vi "Update Waveform Array.vi"(8 "error in (no error)":errorcluster caption="错误输入（无错误）", 10 "new waveform array":waveform(dbl)[](array[waveform]) caption="新波形数组", 11 "original waveform array":waveform(dbl)[](array[waveform]) caption="原波形数组") -> (0 "error out":errorcluster caption="错误输出", 2 "min duration":dbl caption="最小时长", 3 "updated wavefrom array":waveform(dbl)[](array[waveform]) caption="更新后波形数组")   [LabVIEW 2015]
uses:
  <vilib>/Waveform/WDTOps.llb/WDT Index Channel DBL.vi
  <vilib>/Waveform/WDTOps.llb/WDT Append Waveforms DBL.vi
  <vilib>/Waveform/WDTOps.llb/WDT Waveform Duration DBL.vi
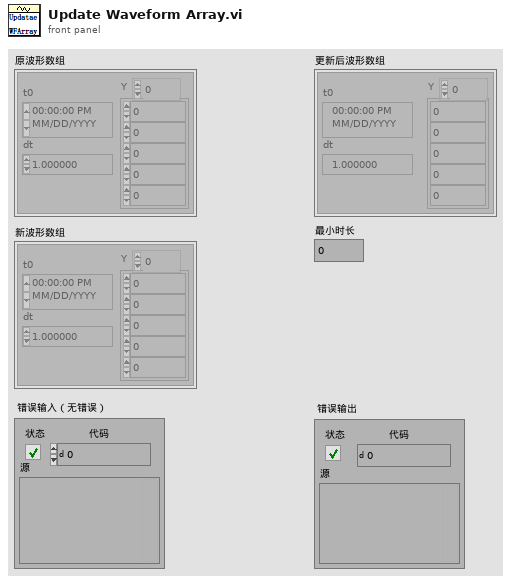
[diagram p1: front panel]
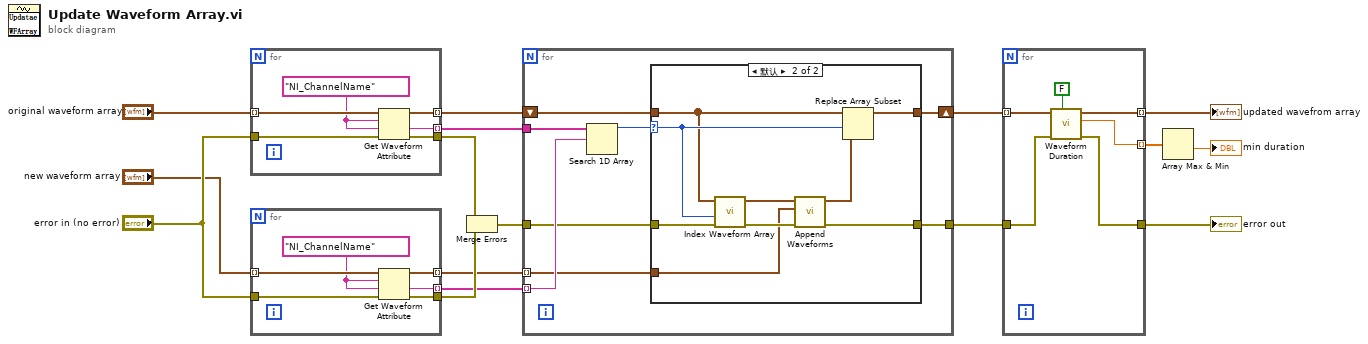
[diagram p0: block diagram]
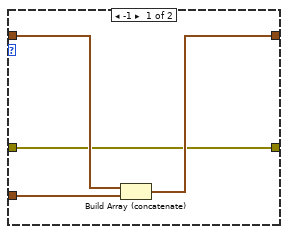
[diagram p2: hidden frame]
diagram:
  n1 = for {
    tunnel: "original waveform array" -> [w22] mode=indexing
    tunnel: "error in (no error)" -> [w21]
    tunnel: [w19] -> w14 mode=indexing
    tunnel: [w18] -> w13 mode=indexing
    tunnel: [w17] -> w11
    w20 = "NI_ChannelName" ("名称")
    n2 = Get Waveform Attribute(4:w21, 5:w20, 6:w20, 7:w22) -> (0:w17:errorcluster, 1:w19:string, 3:w18:waveform(dbl))  [unwired: 1 out]
  }
  n3 = for {
    tunnel: "new waveform array" -> [w28] mode=indexing
    tunnel: "error in (no error)" -> [w27]
    tunnel: [w25] -> w10 mode=indexing
    tunnel: [w24] -> w9 mode=indexing
    tunnel: [w23] -> w12
    w26 = "NI_ChannelName" ("名称")
    n4 = Get Waveform Attribute(4:w27, 5:w26, 6:w26, 7:w28) -> (0:w23:errorcluster, 1:w25:string, 3:w24:waveform(dbl))  [unwired: 1 out]
  }
  n5 = Merge Errors(w11, w12) -> (w8:errorcluster)
  n6 = for {
    tunnel: w14 -> [w36]
    tunnel: w10 -> [w35] mode=indexing
    tunnel: w9 -> [w32] mode=indexing
    shift-right: [w30] -> w7
    shift-left: w13 -> [w31]
    tunnel: w8 -> [w33]
    tunnel: [w29] -> w5
    n7 = Search 1D Array(1D array=w36, element=w35) -> (index of element=w34:i32)  [unwired: 1 in]
    n8 = case shown="默认" w34 {
      selector: w34 -> [_ w45]
      tunnel: w31 -> [w40 w41]
      tunnel: w33 -> [w37 w47]
      tunnel: w32 -> [w39 w46]
      tunnel: [w38 w43] -> w30
      tunnel: [w37 w42] -> w29
      frame -1 {
        n9 = Build Array (concatenate)(w40, w39) -> (w38:waveform(dbl)[])
      }
      frame Default {
        n10 = call-poly <vilib>:"Index Waveform Array.vi"("error in (no error)"=w47, "index"=w45, "waveform array"=w41) -> ("error out"=w48:errorcluster, "waveform"=w49:waveform(dbl))  [unwired: 7 in]
        n11 = call-poly <vilib>:"Append Waveforms.vi"("error in (no error)"=w48, "waveform B"=w46, "waveform A"=w49) -> ("error out"=w42:errorcluster, "waveform out"=w44:waveform(dbl))  [unwired: 7 in]
        n12 = Replace Array Subset(array=w41, new element=w44, index=w45) -> (w43:waveform(dbl)[])
      }
    }
  }
  n13 = for {
    tunnel: w7 -> [w55] mode=indexing
    tunnel: [w54] -> w6 mode=indexing
    tunnel: w5 -> [w53]
    tunnel: [w52] -> w4
    tunnel: [w51] -> w2 mode=indexing
    n14 = call-poly <vilib>:"Waveform Duration.vi"("open interval? (T)"=FALSE, "error in (no error)"=w53, "waveform in"=w55) -> ("error out"=w52:errorcluster, "duration"=w51:dbl, "waveform out"=w54:waveform(dbl))  [unwired: 6 in]
  }
  "error out" <- w4
  "updated wavefrom array" <- w6
  n15 = Array Max & Min(array=w2) -> (min value=→"min duration":dbl)  [unwired: 3 out]
